vi "Read Raw String.vi"(8 "error in (no error)":errorcluster, 11 "Filter Wheel Simulator in":refnum<class "Filter Wheel Simulator.lvclass">) -> (0 "error out":errorcluster, 2 "Raw String":string, 3 "Filter Wheel Simulator out":refnum<class "Filter Wheel Simulator.lvclass">)   [LabVIEW 2024, in "Filter Wheel Simulator.lvclass"]
uses:
  Filter Wheel Simulator.lvclass
  Filter Wheel Simulator.lvclass/Filter Wheel Simulator.ctl
  Filter Wheel Object/Filter Wheel.lvclass
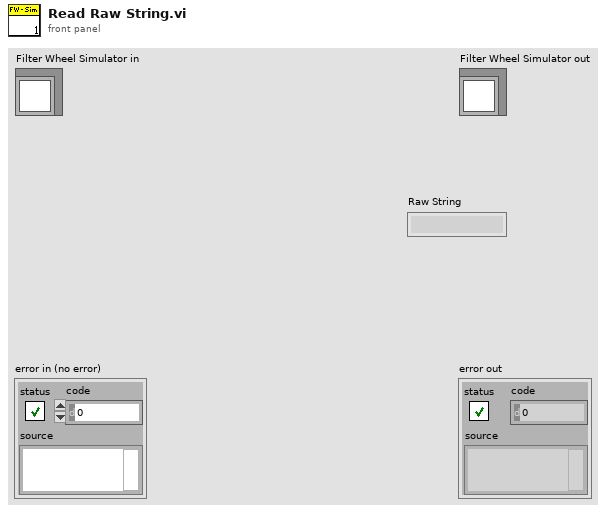
[diagram p1: front panel]
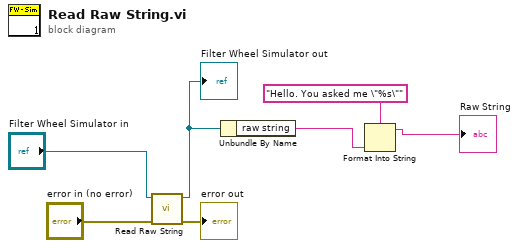
[diagram p0: block diagram]
diagram:
  n1 = call-parent "Read Raw String.vi"("error in (no error)"="error in (no error)", "Filter Wheel in"="Filter Wheel Simulator in") -> ("error out"=→"error out":errorcluster, "Filter Wheel out"=w4:refnum<class "Filter Wheel Simulator.lvclass">)  [unwired: 7 in, 1 out]
  "Filter Wheel Simulator out" <- w4
  n2 = Unbundle By Name(w4) -> ("raw string"=w2:string)
  n3 = Format Into String(format string="Hello. You asked me \"%s\"", w2) -> (resulting string=→"Raw String":string)  [unwired: 2 in, 1 out]
